vi "Read Buffer Data.vi"(8 "error in (no error)":errorcluster, 10 "Storage Type (2:All)":u16(ring)=2 items=["Voltage", "Current", "All"], 11 "VISA resource name":refnum<visa-resource-name>) -> (0 "error out":errorcluster, 2 "Stored Readings":dbl[][](array[numeric]) format="%_5g", 3 "VISA resource name out":refnum<visa-resource-name>)   [LabVIEW 2018, in "BK Precision 8600 Series.lvlib"]
doc: "Reads the stored readings of the selected storage type from buffer storage operation. It returns a 2D-array that contains voltage, current, or voltage and current readings. If storage type is voltage or current, the second column of the array will be all initialized to 0."
uses:
  <instrlib>/BK Precision 8600 Series/BK Precision 8600 Series.lvlib
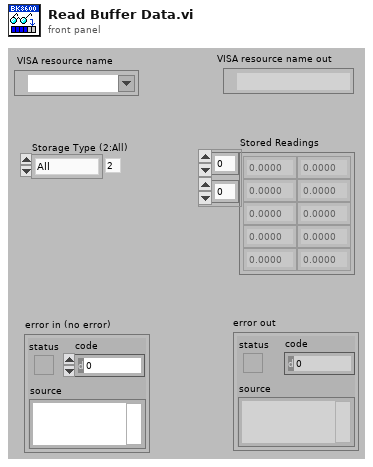
[diagram p1: front panel]
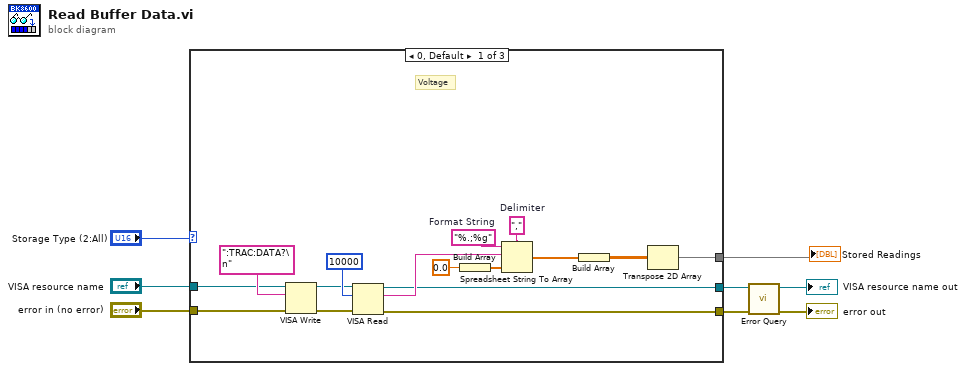
[diagram p0: block diagram]
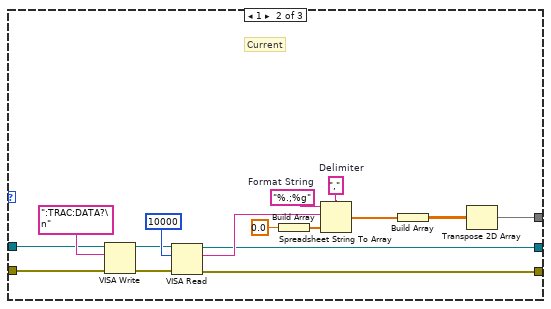
[diagram p2: hidden frame]
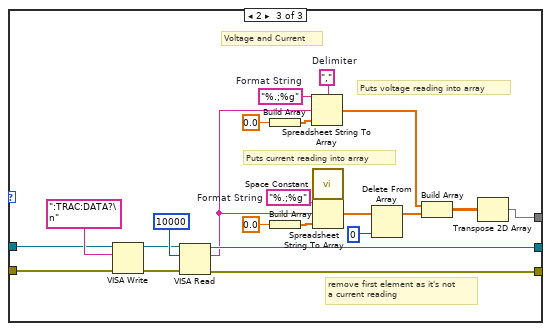
[diagram p3: hidden frame]
diagram:
  n1 = case shown="0, Default" "Storage Type (2:All)" {
    tunnel: "VISA resource name" -> [w16 w32 w49]
    tunnel: "error in (no error)" -> [w15 w31 w48]
    tunnel: [w13 w29 w47] -> w7
    tunnel: [w12 w28 w46] -> w6
    tunnel: [w9 w25 w42] -> w8
    frame 0, Default {
      w21 = ","  # Delimiter
      w24 = "%.;%g"  # Format String
      # "Voltage"
      n2 = VISA Write(VISA resource name=w16, write buffer=":TRAC:DATA?\n", error in (no error)=w15) -> (VISA resource name out=w18:refnum<visa-resource-name>, error out=w17:errorcluster)  [unwired: 1 out]
      n3 = VISA Read(VISA resource name=w18, byte count=10000, error in (no error)=w17) -> (VISA resource name out=w13:refnum<visa-resource-name>, read buffer=w14:string, error out=w12:errorcluster)  [unwired: 1 out]
      n4 = Build Array(0.0) -> (w22:dbl[])
      n5 = Spreadsheet String To Array(delimiter (Tab)=w21, format string=w24, spreadsheet string=w14, array type (2D Dbl)=w22) -> (array=w11:dbl[])
      n6 = Build Array(w11) -> (w10:dbl[][])
      n7 = Transpose 2D Array(2D array=w10) -> (transposed array=w9:dbl[][])
    }
    frame 1 {
      w37 = ","  # Delimiter
      w40 = "%.;%g"  # Format String
      # "Current"
      n8 = VISA Write(VISA resource name=w32, write buffer=":TRAC:DATA?\n", error in (no error)=w31) -> (VISA resource name out=w34:refnum<visa-resource-name>, error out=w33:errorcluster)  [unwired: 1 out]
      n9 = VISA Read(VISA resource name=w34, byte count=10000, error in (no error)=w33) -> (VISA resource name out=w29:refnum<visa-resource-name>, read buffer=w30:string, error out=w28:errorcluster)  [unwired: 1 out]
      n10 = Build Array(0.0) -> (w38:dbl[])
      n11 = Spreadsheet String To Array(delimiter (Tab)=w37, format string=w40, spreadsheet string=w30, array type (2D Dbl)=w38) -> (array=w27:dbl[])
      n12 = Build Array(w27) -> (w26:dbl[][])
      n13 = Transpose 2D Array(2D array=w26) -> (transposed array=w25:dbl[][])
    }
    frame 2 {
      w57 = "%.;%g"  # Format String
      w60 = ","  # Delimiter
      w63 = "%.;%g"  # Format String
      # "remove first element as it's not\na current reading"
      # "Puts current reading into array"
      # "Puts voltage reading into array"
      # "Voltage and Current"
      n14 = VISA Write(VISA resource name=w49, write buffer=":TRAC:DATA?\n", error in (no error)=w48) -> (VISA resource name out=w51:refnum<visa-resource-name>, error out=w50:errorcluster)  [unwired: 1 out]
      n15 = VISA Read(VISA resource name=w51, byte count=10000, error in (no error)=w50) -> (VISA resource name out=w47:refnum<visa-resource-name>, read buffer=w41:string, error out=w46:errorcluster)  [unwired: 1 out]
      n16 = Build Array(0.0) -> (w61:dbl[])
      n17 = Build Array(0.0) -> (w56:dbl[])
      n18 = Spreadsheet String To Array(delimiter (Tab)=w60, format string=w63, spreadsheet string=w41, array type (2D Dbl)=w61) -> (array=w43:dbl[])
      n19 = call <vilib>:"Space Constant.vi"() -> ("String"=w58:string)
      n20 = Spreadsheet String To Array(delimiter (Tab)=w58, format string=w57, spreadsheet string=w41, array type (2D Dbl)=w56) -> (array=w54:dbl[])
      n21 = Delete From Array(array=w54, index=0) -> (array with subset deleted=w44:dbl[])  [unwired: 1 in, 1 out]
      n22 = Build Array(w43, w44) -> (w45:dbl[][])
      n23 = Transpose 2D Array(2D array=w45) -> (transposed array=w42:dbl[][])
    }
  }
  "Stored Readings" <- w8
  n24 = call <instrlib>:"Error Query.vi"("error in (no error)"=w6, "VISA resource name"=w7) -> ("error out"=→"error out":errorcluster, "VISA resource name out"=→"VISA resource name out":refnum<visa-resource-name>)  [unwired: 6 in, 2 out]
